vi "crio_RT_Plant.vi"   [LabVIEW 2019]
uses:
  <vilib>/IEDriver/SPIandI2C/Host/SPI/SPI Host.lvlib
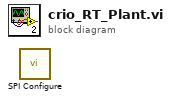
[diagram p0: block diagram]
diagram:
  n1 = call <vilib>:"SPI Configure.vi"() -> ()  [unwired: 14 in, 2 out]
